vi "Read Modulation Envelope Amplitude from State.vi"(8 "error in (no error)":errorcluster, 11 "SV Signal in":refnum<class "SV Signal.lvclass">) -> (0 "error out":errorcluster, 2 "modulation envelope amplitude":dbl=nan, 3 "SV Signal out":refnum<class "SV Signal.lvclass">)   [LabVIEW 2017, in "SV Signal.lvclass"]
uses:
  <vilib>/addons/_NISVFA/_Generation/Signal Generation/SV Signal/SV Signal.lvclass
  <vilib>/addons/_NISVFA/_Generation/Signal Generation/SV Signal/SV Signal.lvclass/SV Signal.ctl
  <vilib>/addons/_NISVFA/_Generation/Signal Generation/SV Signal/sv_Signal State Attribute.ctl
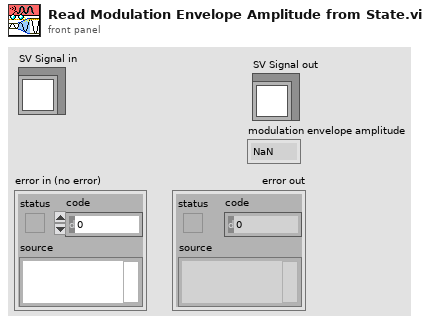
[diagram p1: front panel]
types:
  T1 = typedef "SV Signal.lvclass/sv_Signal State Attribute.ctl" = string
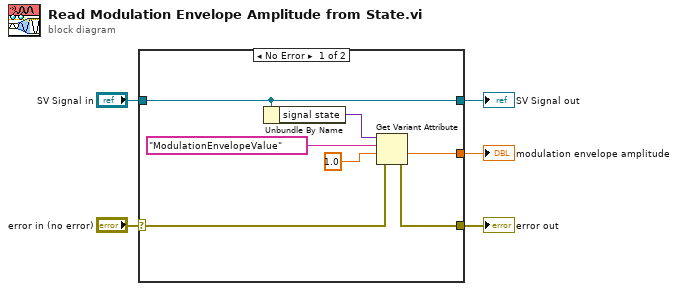
[diagram p0: block diagram]
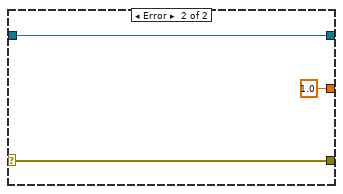
[diagram p2: hidden frame]
diagram:
  n1 = case shown="No Error" "error in (no error)" {
    selector: "error in (no error)" -> [w6 w15]
    tunnel: [w10 w15] -> w5
    tunnel: [w8 1.0 ("amplitude")] -> w4
    tunnel: "SV Signal in" -> [w7 w14]
    tunnel: [w7 w14] -> w2
    frame No Error {
      n2 = Unbundle By Name(w7) -> ("signal state"=w11:variant)
      n3 = Get Variant Attribute(Variant=w11, name=T1 "ModulationEnvelopeValue", default value (empty Variant)=1.0 ("amplitude"), error in=w6) -> (value=w8:dbl, error out=w10:errorcluster)  [unwired: 2 out]
    }
    frame Error {
    }
  }
  "modulation envelope amplitude" <- w4
  "SV Signal out" <- w2
  "error out" <- w5
